vi "eMMcTest.vi"(8 "error in (no error)":errorcluster, 10 "method":string, 11 "Sequence Context In":refnum<k7>) -> (0 "error out":errorcluster, 2 "status":string)   [LabVIEW 2021]
uses:
  <vilib>/addons/TestStand/_TSUtility.llb/TestStand - Get Property Value (String).vi
  <vilib>/NI/JSON Support for LabVIEW/JSON Value/New JSON Value/New JSON ([]).vi
  <vilib>/NI/NI JSONRPC Server Framework/Classes/Client/Format Client Request (Auto-Increment).vi
  <vilib>/NI/JSON Support for LabVIEW/JSON Value/JSON Value.lvclass
  <vilib>/NI/NI JSONRPC Server Framework/Classes/Client/JSONRPC Client.lvclass
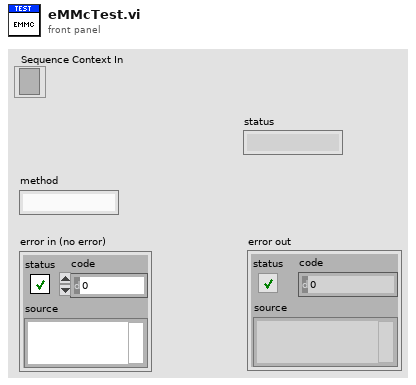
[diagram p1: front panel]
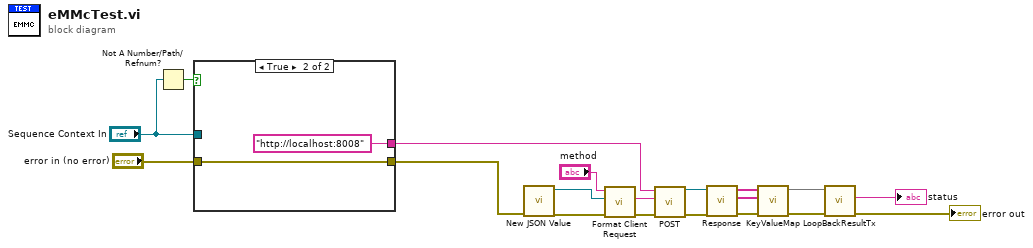
[diagram p0: block diagram]
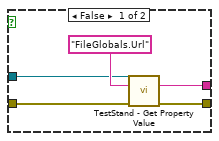
[diagram p2: hidden frame]
diagram:
  n1 = Not A Number/Path/Refnum?(number/path/refnum="Sequence Context In") -> (NaN/Path/Refnum?=w1:bool)
  n2 = case shown="True" w1 {
    tunnel: [w23 "http://localhost:8008" ("Value")] -> w19
    tunnel: [w22 w26] -> w18
    tunnel: "error in (no error)" -> [w21 w26]
    tunnel: "Sequence Context In" -> [w20 _]
    frame False {
      n3 = call-poly <vilib>:"TestStand - Get Property Value.vi"("Sequence Context In"=w20, "Lookup String"="FileGlobals.Url", "error in (no error)"=w21) -> ("Value"=w23:string, "error out"=w22:errorcluster)  [unwired: 10 in, 1 out]
    }
    frame True {
    }
  }
  n4 = call-poly <vilib>:"New JSON Value.vi"("error in (no error)"=w18) -> ("error out"=w7:errorcluster, "JSON Value out"=w6:refnum<class "JSON Value.lvclass">)  [unwired: 9 in]
  n5 = call-poly <vilib>:"Format Client Request.vi"("error in (no error)"=w7, "JSON Value in"=w6, "method"="method") -> ("error out"=w9:errorcluster, "Request String"=w10:string)  [unwired: 7 in]
  n6 = call "POST.vi"("error in (no error)"=w9, "Request String"=w10, "url"=w19) -> ("error out"=w11:errorcluster, "JSON Value out"=w12:refnum<class "JSON Value.lvclass">)  [unwired: 7 in]
  n7 = call "Response.vi"("error in (no error)"=w11, "JSON Value in"=w12) -> ("error out"=w13:errorcluster, "values"=w15:string[], "keys"=w14:string[])  [unwired: 7 in]
  n8 = call "KeyValueMap.vi"("error in"=w13, "values"=w15, "keys"=w14) -> ("error out"=w4:errorcluster, "map out"=w5:map{string, string})  [unwired: 7 in]
  n9 = call "LoopBackResultTx.vi"("error in (no error)"=w4, "map"=w5) -> ("error out"=→"error out":errorcluster, "status"=→"status":string)  [unwired: 8 in]
